vi "T Test (2-sample).vi"(6 "alternative hypothesis":i32(ring) items=["mean(x) != mean(y)"=0, "mean(x) > mean(y)"=1, "mean(x) < mean(y)"=-1], 9 "significance level":dbl=0.05, 10 "sample set y":dbl[](array[numeric]), 11 "sample set x":dbl[](array[numeric])) -> (0 "error":i32, 1 "confidence interval":cluster{"low":dbl, "high":dbl}={"low"=0.8260722090132093, "high"=0.8260722090132093} {"high" format="%.6g"; "low" format="%.6g"}, 2 "p value":dbl=0.05 format="%.6g", 3 "reject null hypothesis":bool, 4 "t test info":T1 {"sample t value" format="%_6g"; "t value" format="%_6g"; "sample se mean" format="%_6g"; "sample std" format="%_6g"; "sample mean" format="%_6g"})   [LabVIEW 2010, in "NI_Gmath.lvlib"]
doc: "See pages 278+ from Applied Statistics and Probability for Engineers (Montgomery) - 3rd Edition."
uses:
  NI_Gmath.lvlib
  st_t_control.ctl
  NI_AALBase.lvlib
panel:
  # "T Test\n(two sample sets)"
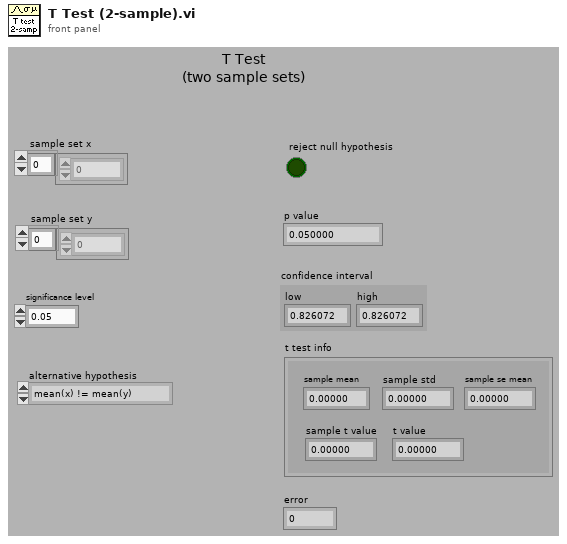
[diagram p1: front panel]
types:
  T1 = typedef "NI_Gmath.lvlib/st_t_control.ctl" = cluster{"sample mean":dbl, "sample std":dbl, "sample se mean":dbl, "sample t value":dbl, "t value":dbl}
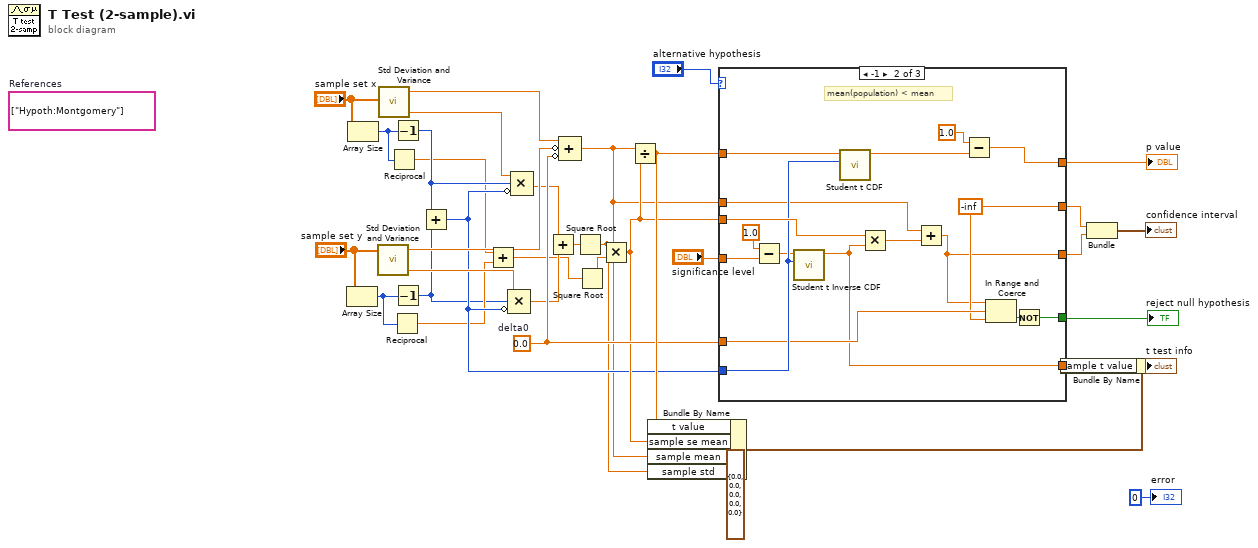
[diagram p0: block diagram]
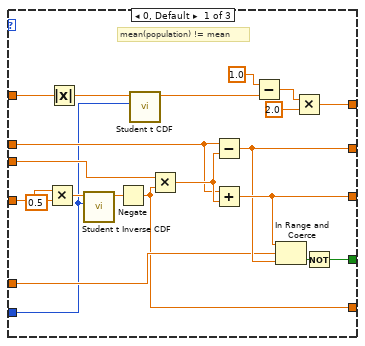
[diagram p2: hidden frame]
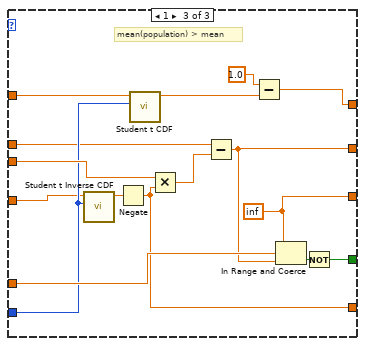
[diagram p3: hidden frame]
diagram:
  w19 = 0.0  # delta0
  (unwired) string[] ["Hypoth:Montgomery"]  # References
  n1 = Array Size(array="sample set y") -> (size(s)=w13:i32)
  n2 = Array Size(array="sample set x") -> (size(s)=w11:i32)
  n3 = call "Std Deviation and Variance.vi"("X"="sample set y") -> ("mean"=w20:dbl, "variance"=w18:dbl)  [unwired: 1 in, 1 out]
  n4 = call "Std Deviation and Variance.vi"("X"="sample set x") -> ("mean"=w28:dbl, "variance"=w3:dbl)  [unwired: 1 in, 1 out]
  n5 = Reciprocal(x=w11) -> (1/x=w9:dbl)
  n6 = Reciprocal(x=w13) -> (1/x=w10:dbl)
  n7 = Decrement(x=w11) -> (x-1=w12:i32)
  n8 = Decrement(x=w13) -> (x-1=w2:i32)
  n9 = Add(x=w12, y=w2) -> (x+y=w14:i32)
  n10 = Add(x=w9, y=w10) -> (x+y=w6:dbl)
  n11 = Compound Arithmetic op=MULTIPLY(w18, w2, invert w14) -> (w16:dbl)
  n12 = Compound Arithmetic op=MULTIPLY(w3, w12, invert w14) -> (w17:dbl)
  n13 = Add(x=w17, y=w16) -> (x+y=w8:dbl)
  n14 = Compound Arithmetic op=ADD(w28, invert w20, invert w19) -> (w1:dbl)
  n15 = Square Root(x=w8) -> (sqrt(x)=w5:dbl)
  n16 = Square Root(x=w6) -> (sqrt(x)=w7:dbl)
  n17 = Multiply(x=w5, y=w7) -> (x*y=w15:dbl)
  n18 = Divide(x=w1, y=w15) -> (x/y=w27:dbl)
  n19 = Bundle By Name(cluster=T1 {"sample mean"=0.0, "sample std"=0.0, "sample se mean"=0.0, "sample t value"=0.0, "t value"=0.0} ("t test info"), "t value"=w27, "sample se mean"=w15, "sample mean"=w1, "sample std"=w5) -> (w26:T1)
  n20 = case shown="-1" "alternative hypothesis" {
    tunnel: "significance level" -> [w55 w62 w80]
    tunnel: w14 -> [w44 w69 w84]
    tunnel: w15 -> [w54 w73 w89]
    tunnel: [w50 w57 w77] -> w32
    tunnel: [w49 w58 w78] -> w31
    tunnel: [w47 w70 w86] -> w4
    tunnel: w19 -> [w46 w65 w85]
    tunnel: w1 -> [w45 w64 w79]
    tunnel: w27 -> [w43 w59 w83]
    tunnel: [w38 w66 w76] -> w29
    tunnel: [w37 w60 w74] -> w24
    frame 0, Default {
      # "mean(population) != mean"
      n21 = Multiply(x=w55, y=0.5) -> (x*y=w51:dbl)
      n22 = Absolute Value(x=w43) -> (abs(x)=w36:dbl)
      n23 = call "Student t Inverse CDF.vi"("k degrees of freedom"=w44, "cdf(x)"=w51) -> ("x"=w52:dbl)  [unwired: 8 in, 1 out]
      n24 = Negate(x=w52) -> (-x=w37:dbl)
      n25 = call "Student t CDF.vi"("k degrees of freedom"=w44, "x"=w36) -> ("cdf(x)"=w41:dbl)  [unwired: 7 in, 2 out]
      n26 = Multiply(x=w54, y=w37) -> (x*y=w53:dbl)
      n27 = Subtract(x=w45, y=w53) -> (x-y=w49:dbl)
      n28 = Add(x=w45, y=w53) -> (x+y=w50:dbl)
      n29 = Subtract(x=1.0, y=w41) -> (x-y=w39:dbl)
      n30 = In Range and Coerce(upper limit=w50, x=w46, lower limit=w49) -> (In Range?=w48:bool)  [unwired: 1 out]
      n31 = Multiply(x=w39, y=2.0) -> (x*y=w38:dbl)
      n32 = Not(x=w48) -> (.not. x?=w47:bool)
    }
    frame -1 {
      w58 = -inf ("lower limit")
      # "mean(population) < mean"
      n33 = Subtract(x=1.0, y=w62) -> (x-y=w61:dbl)
      n34 = call "Student t Inverse CDF.vi"("k degrees of freedom"=w69, "cdf(x)"=w61) -> ("x"=w60:dbl)  [unwired: 8 in, 1 out]
      n35 = call "Student t CDF.vi"("k degrees of freedom"=w69, "x"=w59) -> ("cdf(x)"=w67:dbl)  [unwired: 7 in, 2 out]
      n36 = Multiply(x=w73, y=w60) -> (x*y=w72:dbl)
      n37 = Add(x=w64, y=w72) -> (x+y=w57:dbl)
      n38 = Subtract(x=1.0, y=w67) -> (x-y=w66:dbl)
      n39 = In Range and Coerce(upper limit=w57, x=w65, lower limit=w58) -> (In Range?=w71:bool)  [unwired: 1 out]
      n40 = Not(x=w71) -> (.not. x?=w70:bool)
    }
    frame 1 {
      w77 = inf
      # "mean(population) > mean"
      n41 = call "Student t Inverse CDF.vi"("k degrees of freedom"=w84, "cdf(x)"=w80) -> ("x"=w75:dbl)  [unwired: 8 in, 1 out]
      n42 = Negate(x=w75) -> (-x=w74:dbl)
      n43 = call "Student t CDF.vi"("k degrees of freedom"=w84, "x"=w83) -> ("cdf(x)"=w81:dbl)  [unwired: 7 in, 2 out]
      n44 = Multiply(x=w89, y=w74) -> (x*y=w88:dbl)
      n45 = Subtract(x=w79, y=w88) -> (x-y=w78:dbl)
      n46 = Subtract(x=1.0, y=w81) -> (x-y=w76:dbl)
      n47 = In Range and Coerce(upper limit=w77, x=w85, lower limit=w78) -> (In Range?=w87:bool)  [unwired: 1 out]
      n48 = Not(x=w87) -> (.not. x?=w86:bool)
    }
  }
  "reject null hypothesis" <- w4
  "p value" <- w29
  n49 = Bundle By Name(cluster=w26, "sample t value"=w24) -> (→"t test info":T1)
  n50 = Bundle("lower limit"=w31, w32) -> (→"confidence interval":cluster{"lower limit":dbl, dbl})  [unwired: 1 in]
  "error" <- 0 ("error")
